vi "basic - Transmit and Update (from FIle).vi"() -> ()   [LabVIEW 2020]
doc: "Overview: Setup the board to transmit package as raw frames.\nRequirement: One AIM ARINC-664 board with installed AIM ARINC 664 BSP.\nRestrictions: None.\nInstruction:\n1. Select the Board ID (0 if you have only one board in your system) and the port number. If you want to validate between two ports in one device, you can use tx board and Rx Board\n2. Run the VI.\n3. See the result in the Indicators and press STOP to stop the VI.s\nFor detailed information about functions use, see documents in <BSP Installation folder>\\AIM GmbH\\Arinc 664 Windows BSP <version>\\Doc."
uses:
  Frame Configuration/controls/frame_file_entry.ctl
  Frame Configuration/controls/frame_record_type.ctl
  <instrlib>/AIM GmbH/_AIM 664/_controls/queue_header_generic.ctl
  <instrlib>/AIM GmbH/_AIM 664/bsp/Fdx Create Session (Tx-Generic).vi
  <instrlib>/AIM GmbH/_AIM 664/bsp/Fdx Start (Tx).vi
  <instrlib>/AIM GmbH/_AIM 664/bsp/Fdx Stop (Tx).vi
  <instrlib>/AIM GmbH/_AIM 664/AIM664LV.lvlib
panel:
  out "Array":cluster{"frame size":i32, "payload size":i32}[](array[cluster])
  in  "QueueSizeIn":u32
  in  "Index":u32
  in  "value.Data":u8[](array[numeric]) format="%.0x"
  out "exec time uS":u32
  in  "update":bool
  out "data":T1[](array[typedef]) {"value"."Data" format="%.0x"; "value"."HeaderInfo"."NetSelect" items=["FDX_TX_FRAME_DLY_A"=0, "FDX_TX_FRAME_DLY_B"=1, "FDX_TX_FRAME_BOTH "=3, "FDX_TX_FRAME_ONLY_A"=4, "FDX_TX_FRAME_ONLY_B "=5]; "value"."HeaderInfo"."FrameStartMode" items=["FDX_TX_FRAME_START_IFG", "FDX_TX_FRAME_START_PGWT", "FDX_TX_FRAME_START_TRG"]; "value"."HeaderInfo"."PhysErrorInjection" items=["FDX_TX_FRAME_ERR_OFF"=0, "FDX_TX_FRAME_ERR_CRC"=1, "FDX_TX_FRAME_ERR_ALI"=2, "FDX_TX_FRAME_ERR_PRE"=4, "FDX_TX_FRAME_ERR_PHY"=8]; "value"."HeaderInfo"."SequenceNumberInit" items=["FDX_TX_FRAME_SEQ_INIT_AUTO"=65535]; "value"."HeaderInfo"."SequenceNumberOffset" items=["FDX_TX_FRAME_SEQ_OFFS_AUTO "=65535]; "value"."HeaderInfo"."PayloadGenerationMode" items=["FDX_TX_FRAME_PGM_USER"=0, "FDX_TX_FRAME_PGM_IP_PART"=1, "FDX_TX_FRAME_PGM_IP_FULL"=2, "FDX_TX_FRAME_PGM_IP_PART_TT"=10, "FDX_TX_FRAME_PGM_IP_FULL_TT"=20]; "value"."HeaderInfo"."PayloadBufferMode" items=["FDX_TX_FRAME_PBM_STD", "FDX_TX_FRAME_PBM_MAC", "FDX_TX_FRAME_PBM_UDP"]}
  in  "file path (use dialog)":path=path "/home/lvuser/standard_frames_udp_v1.bin"
  in  "PortMap":u32
  out "Duplicated":bool
  out "TxStatus":T4={"TxStatus"=1, "Frames"=855, "TransmitMode"=0, "FramesPortB"=0}
  out "TxQueueStatus":T5={"QueueStatus"=0, "BytesReloadable"=0, "FramesSent"=854, "FramesInCycQueue"=0} {"QueueStatus" items=["FDX_QUE_EMPTY", "FDX_QUE_FILLED", "FDX_QUE_FULL", "FDX_QUE_SENT", "FDX_QUE_CYCL_RUN", "FDX_QUE_CYCL_SENT"]}
  out "TxQueueInfo":cluster{"QueueBaseAddr":u32, "QueueSizeOut":u32}={"QueueBaseAddr"=50892800, "QueueSizeOut"=4194304}
  in  "Port":u32
  in  "Board":u32
  out "current time":timestamp=timestamp(3686777794.875688 s since 1904-01-01)
  out "current irig time":T6={"SignOut"=40, "DayOut"=1, "HourOut"=1, "MinOut"=28, "SecondOut"=39, "MilliSecOut"=539, "MicroSecOut"=300, "NanoSecOut"=0, "InfoOut"=0, "Mode"=3}
  in  "stop":bool
  out "PortInitOut":T7={"PortConfig"=0, "PortUsed"=1, "GlobalMemFree"=0, "SharedMemFree"=0} {"PortConfig" items=["FDX_SINGLE", "FDX_REDUNDANT"]}
  out "error out":errorcluster
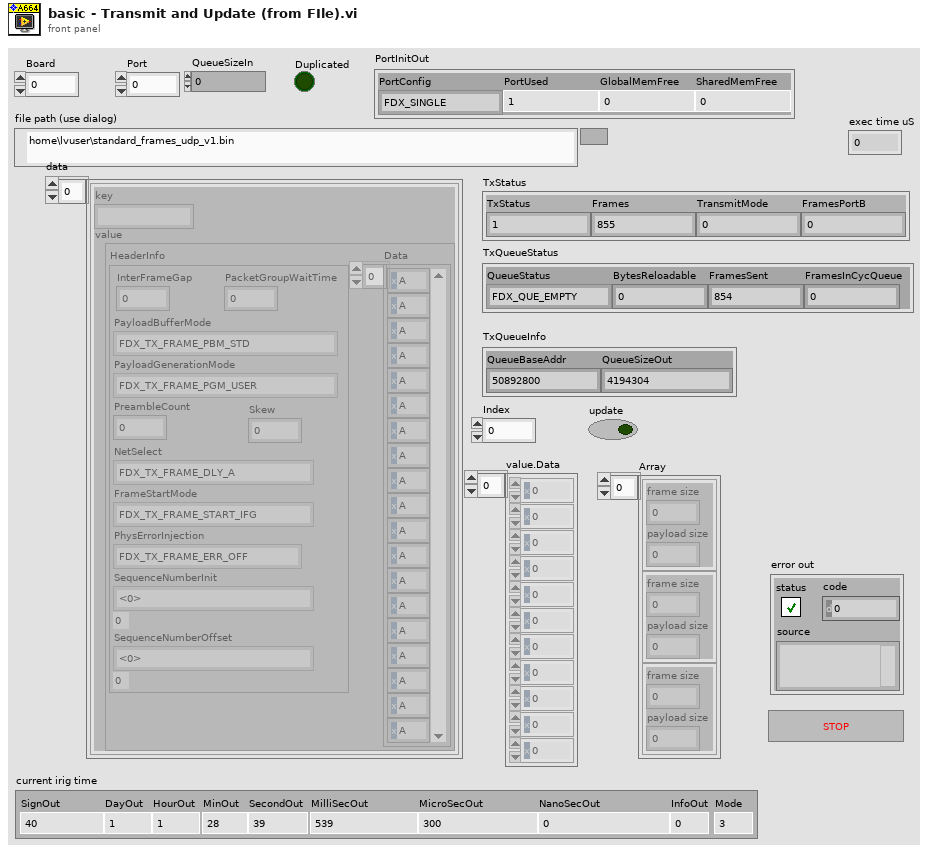
[diagram p1: front panel]
types:
  T1 = typedef "frame_file_entry.ctl" = cluster{"key":string, "value":T2}
  T2 = typedef "frame_record_type.ctl" = cluster{"HeaderInfo":T3, "Data":u8[]}
  T3 = typedef "AIM664LV.lvlib/queue_header_generic.ctl" = cluster{"InterFrameGap":u32, "PacketGroupWaitTime":u32, "PayloadBufferMode":u8, "PayloadGenerationMode":u8, "PreambleCount":u8, "Skew":u32, "NetSelect":u8, "FrameStartMode":u8, "PhysErrorInjection":u32, "SequenceNumberInit":u16, "SequenceNumberOffset":u16}
  T4 = cluster{"TxStatus":u32, "Frames":u32, "TransmitMode":u32, "FramesPortB":u32}
  T5 = cluster{"QueueStatus":i32, "BytesReloadable":u32, "FramesSent":u32, "FramesInCycQueue":u32}
  T6 = cluster{"SignOut":i32, "DayOut":u32, "HourOut":u32, "MinOut":u32, "SecondOut":u32, "MilliSecOut":u32, "MicroSecOut":u32, "NanoSecOut":u32, "InfoOut":u32, "Mode":u32}
  T7 = cluster{"PortConfig":u32, "PortUsed":u32, "GlobalMemFree":u32, "SharedMemFree":u32}
  T8 = cluster{"Index":u32, "Offset":u32, "Length":u32, "SubQueueHandle":u32}
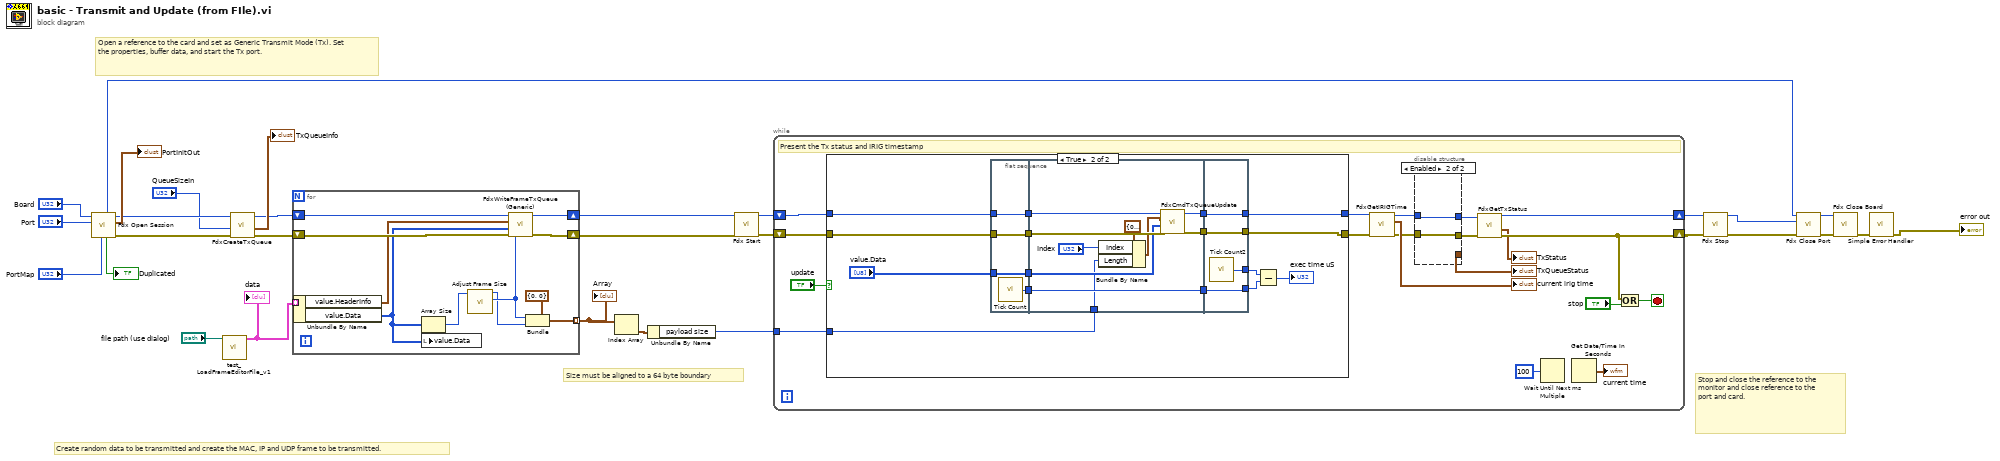
[diagram p0: block diagram]
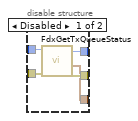
[diagram p2: hidden frame]
diagram:
  # "Size must be aligned to a 64 byte boundary"
  # "Stop and close the reference to the monitor and close reference to the port and card."
  # "Create random data to be transmitted and create the MAC, IP and UDP frame to be transmitted."
  # "Open a reference to the card and set as Generic Transmit Mode (Tx). Set the properties, buffer data, and start the Tx port."
  n1 = call-poly <instrlib>:"Fdx Open Session.vi"("PortMap"="PortMap", "port"="Port", "board"="Board") -> ("error out"=w23:errorcluster, "PortInitOut"=→"PortInitOut":T7, "port handle out"=w24:u32, "Duplicated"=→"Duplicated":bool, "InstrumentHandle_board out"=w12:u32)  [unwired: 3 in, 1 out]
  n2 = call "test_LoadFrameEditorFile_v1.vi"("BIN file path"="file path (use dialog)") -> ("data"=w6:T1[])  [unwired: 9 in, 1 out]
  "data" <- w6
  n3 = call <instrlib>:"FdxCreateTxQueue.vi"("error in"=w23, "QueueSizeIn"="QueueSizeIn", "InstrumentHandle_port"=w24) -> ("error out"=w21:errorcluster, "TxQueueInfo"=→"TxQueueInfo":cluster{"QueueBaseAddr":u32, "QueueSizeOut":u32}, "InstrumentHandle_port"=w19:u32)  [unwired: 6 in]
  n4 = for {
    shift-right: [w40] -> w5
    shift-left: w21 -> [w41]
    shift-right: [w39] -> w20
    shift-left: w19 -> [w38]
    tunnel: w6 -> [w37] mode=indexing
    tunnel: [w34] -> w3 mode=indexing
    n5 = Unbundle By Name(w37) -> ("value.HeaderInfo"=w36:T3, "value.Data"=w35:u8[])
    n6 = Array Size(array=w35) -> (size(s)=w32:i32)
    n7 = local write "value.Data"(w35) -> ()
    n8 = call "Adjust Frame Size.vi"("original size in"=w32) -> ("adjusted size"=w31:i32, "original size out"=w30:i32)  [unwired: 8 in, 1 out]
    n9 = call <instrlib>:"FdxWriteFrameTxQueue (Generic).vi"("Frame Size"=w31, "error in (no error)"=w41, "Frame in"=w35, "HeaderInfo"=w36, "InstrumentHandle_port in"=w38) -> ("error out"=w40:errorcluster, "InstrumentHandle_port out"=w39:u32)  [unwired: 5 in]
    n10 = Bundle(cluster=cluster{"frame size":i32, "payload size":i32} {"frame size"=0, "payload size"=0}, "frame size"=w31, "payload size"=w30) -> (w34:cluster{"frame size":i32, "payload size":i32})
  }
  "Array" <- w3
  n11 = Index Array(array=w3) -> (element=w2:cluster{"frame size":i32, "payload size":i32})  [unwired: 1 in]
  n12 = Unbundle By Name(w2) -> ("payload size"=w1:i32)
  n13 = call-poly <instrlib>:"Fdx Start.vi"("error in"=w5, "InstrumentHandle_port in"=w20) -> ("error out"=w28:errorcluster, "InstrumentHandle_port out"=w27:u32)  [unwired: 8 in]
  n14 = while {
    shift-right: [w50] -> w17
    shift-left: w27 -> [w47]
    shift-right: [w51] -> w18
    shift-left: w28 -> [w46]
    tunnel: w1 -> [w42]
    stop <- w59 stop-if-true
    # "Present the Tx status and IRIG timestamp"
    n15 = case shown="True" "update" {
      tunnel: w47 -> [w69 w82]
      tunnel: w46 -> [w68 w75]
      tunnel: [w69 w85] -> w44
      tunnel: [w68 w73] -> w43
      tunnel: w42 -> [_ w70]
      frame False {
      }
      frame True {
        n16 = flat-sequence {
          tunnel: [w89] -> w83
          tunnel: w82 -> [w89]
          tunnel: [w88] -> w81
          tunnel: w75 -> [w88]
          tunnel: [w87] -> w79
          tunnel: [w86] -> w72
          tunnel: "value.Data" -> [w86]
          tunnel: [w97] -> w84
          tunnel: w83 -> [w98]
          tunnel: w81 -> [w96]
          tunnel: [w99] -> w80
          tunnel: w79 -> [w99]
          tunnel: [w95] -> w74
          tunnel: w72 -> [w91]
          tunnel: w70 -> [w90]
          tunnel: [w103] -> w85
          tunnel: w84 -> [w103]
          tunnel: [w102] -> w78
          tunnel: [w101] -> w77
          tunnel: w80 -> [w101]
          tunnel: w74 -> [w100]
          tunnel: [w100] -> w73
          frame #0 {
            n17 = call "Tick Count"() -> ("Tick Count(uSec)"=w87:u32)
          }
          frame #1 {
            n18 = Bundle By Name(cluster=T8 {"Index"=0, "Offset"=0, "Length"=0, "SubQueueHandle"=0} ("TxQueueUpdateIn"), "Index"="Index", "Length"=w90) -> (w93:T8)
            n19 = call <instrlib>:"FdxCmdTxQueueUpdate.vi"("error in"=w96, "WriteBuffer"=w91, "TxQueueUpdateIn"=w93, "InstrumentHandle"=w98) -> ("error out"=w95:errorcluster, "InstrumentHandle"=w97:u32)  [unwired: 6 in]
          }
          frame #2 {
            n20 = call "Tick Count2"() -> ("Tick Count(uSec)"=w102:u32)
          }
        }
        n21 = Subtract(x=w78, y=w77) -> (x-y=→"exec time uS":u32)
      }
    }
    n22 = call <instrlib>:"FdxGetIRIGTime.vi"("error in"=w43, "InstrumentHandle_board in"=w44) -> ("error out"=w54:errorcluster, "Curent Irig Time"=→"current irig time":T6, "InstrumentHandle_board out"=w55:u32)  [unwired: 7 in]
    n23 = disable-structure shown="Enabled" {
      disable-tunnel: w55 -> [w65 w66]
      disable-tunnel: w54 -> [w64 w67]
      disable-tunnel: [w63 w66] -> w53
      disable-tunnel: [w62 w67] -> w52
      disable-tunnel: [w61 _] -> w49
      frame Disabled {
        n24 = call <instrlib>:"FdxGetTxQueueStatus.vi"("error in"=w64, "InstrumentHandle"=w65) -> ("error out"=w62:errorcluster, "TxQueueStatus"=w61:T5, "InstrumentHandle"=w63:u32)  [unwired: 7 in]
      }
      frame Enabled {
      }
    }
    "TxQueueStatus" <- w49
    n25 = call <instrlib>:"FdxGetTxStatus.vi"("error in"=w52, "InstrumentHandle_port"=w53) -> ("error out"=w51:errorcluster, "TxStatus"=→"TxStatus":T4, "InstrumentHandle_port"=w50:u32)  [unwired: 7 in]
    n26 = Wait Until Next ms Multiple(millisecond multiple=u32 100) -> ()  [unwired: 1 out]
    n27 = Get Date/Time In Seconds() -> (seconds since 1Jan1904=→"current time":timestamp)
    n28 = Or(x=w51, y="stop") -> (x .or. y?=w59:bool)
  }
  n29 = call-poly <instrlib>:"Fdx Stop.vi"("error in"=w18, "InstrumentHandle_port in"=w17) -> ("error out"=w25:errorcluster, "InstrumentHandle_port out"=w14:u32)  [unwired: 8 in]
  n30 = call <instrlib>:"Fdx Close Port.vi"("error in"=w25, "InstrumentHandle_port in"=w14, "InstrumentHandle_board in"=w12) -> ("error out"=w11:errorcluster, "InstrumentHandle_board out"=w8:u32)  [unwired: 7 in]
  n31 = call <instrlib>:"Fdx Close Board.vi"("error in"=w11, "InstrumentHandle_board in"=w8) -> ("error out"=w9:errorcluster)  [unwired: 9 in]
  n32 = call <vilib>:"Simple Error Handler.vi"("error in (no error)"=w9) -> ("error out"=→"error out":errorcluster)  [unwired: 4 in, 4 out]
